vi "GlobalDevice.vi"() -> ()   [LabVIEW 2011]
panel:
  in  "Device Choser":enum32{"Scanner", "Mirror"}(radio)
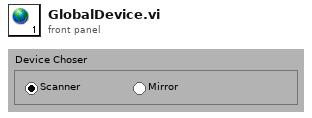
[diagram p1: front panel]
diagram:
